vi "仁科参数写入.vi"(11 "簇":T1 {"时间 16"."分钟" format="%.0f分"; "时间 16"."小时" format="%.0f点"; "时间 15"."分钟" format="%.0f分"; "时间 15"."小时" format="%.0f点"; "时间 14"."分钟" format="%.0f分"; "时间 14"."小时" format="%.0f点"; "时间 13"."分钟" format="%.0f分"; "时间 13"."小时" format="%.0f点"; "时间 12"."分钟" format="%.0f分"; "时间 12"."小时" format="%.0f点"; "时间 11"."分钟" format="%.0f分"; "时间 11"."小时" format="%.0f点"; "时间 10"."分钟" format="%.0f分"; "时间 10"."小时" format="%.0f点"; "时间 9"."分钟" format="%.0f分"; "时间 9"."小时" format="%.0f点"; "时间 8"."分钟" format="%.0f分"; "时间 8"."小时" format="%.0f点"; "时间 7"."分钟" format="%.0f分"; "时间 7"."小时" format="%.0f点"; "时间 6"."分钟" format="%.0f分"; "时间 6"."小时" format="%.0f点"; "时间 5"."分钟" format="%.0f分"; "时间 5"."小时" format="%.0f点"; "时间 4"."分钟" format="%.0f分"; "时间 4"."小时" format="%.0f点"; "时间 3"."分钟" format="%.0f分"; "时间 3"."小时" format="%.0f点"; "时间 2"."分钟" format="%.0f分"; "时间 2"."小时" format="%.0f点"; "时间"."分钟" format="%.0f分"; "时间"."小时" format="%.0f点"}) -> (2 "error out":errorcluster)   [LabVIEW 2016, in "环境动力监测库.lvlib" / "空调库.lvlib"]
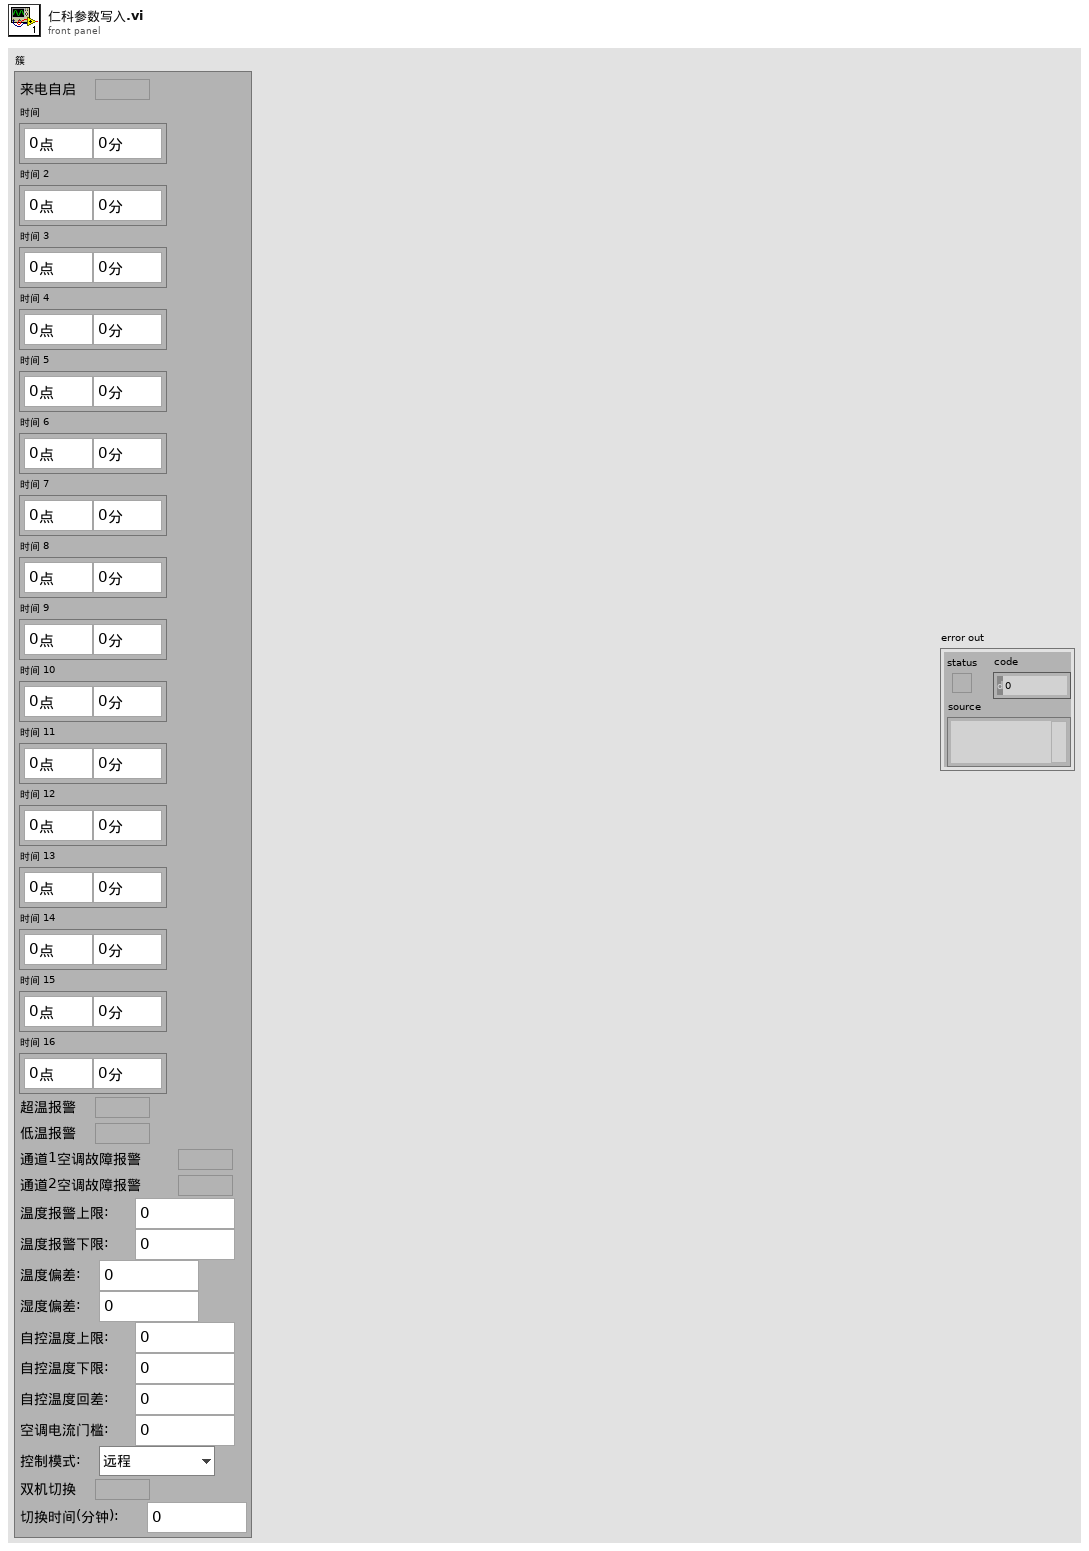
[diagram p1: front panel]
types:
  T1 = cluster{"来电自启":bool, "时间":cluster{"小时":u16, "分钟":u16}, "时间 2":cluster{"小时":u16, "分钟":u16}, "时间 3":cluster{"小时":u16, "分钟":u16}, "时间 4":cluster{"小时":u16, "分钟":u16}, "时间 5":cluster{"小时":u16, "分钟":u16}, "时间 6":cluster{"小时":u16, "分钟":u16}, "时间 7":cluster{"小时":u16, "分钟":u16}, "时间 8":cluster{"小时":u16, "分钟":u16}, "时间 9":cluster{"小时":u16, "分钟":u16}, "时间 10":cluster{"小时":u16, "分钟":u16}, "时间 11":cluster{"小时":u16, "分钟":u16}, "时间 12":cluster{"小时":u16, "分钟":u16}, "时间 13":cluster{"小时":u16, "分钟":u16}, "时间 14":cluster{"小时":u16, "分钟":u16}, "时间 15":cluster{"小时":u16, "分钟":u16}, "时间 16":cluster{"小时":u16, "分钟":u16}, "超温报警":bool, "低温报警":bool, "通道1空调故障报警":bool, "通道2空调故障报警":bool, "温度报警上限:":dbl, "温度报警下限:":dbl, "温度偏差:":dbl, "湿度偏差:":dbl, "自控温度上限:":dbl, "自控温度下限:":dbl, "自控温度回差:":dbl, "空调电流门槛:":dbl, "控制模式:":enum16{"远程", "自动"}, "双机切换":bool, "切换时间(分钟):":dbl}
  T2 = enum16{"open", "read", "write single", "write", "close"}
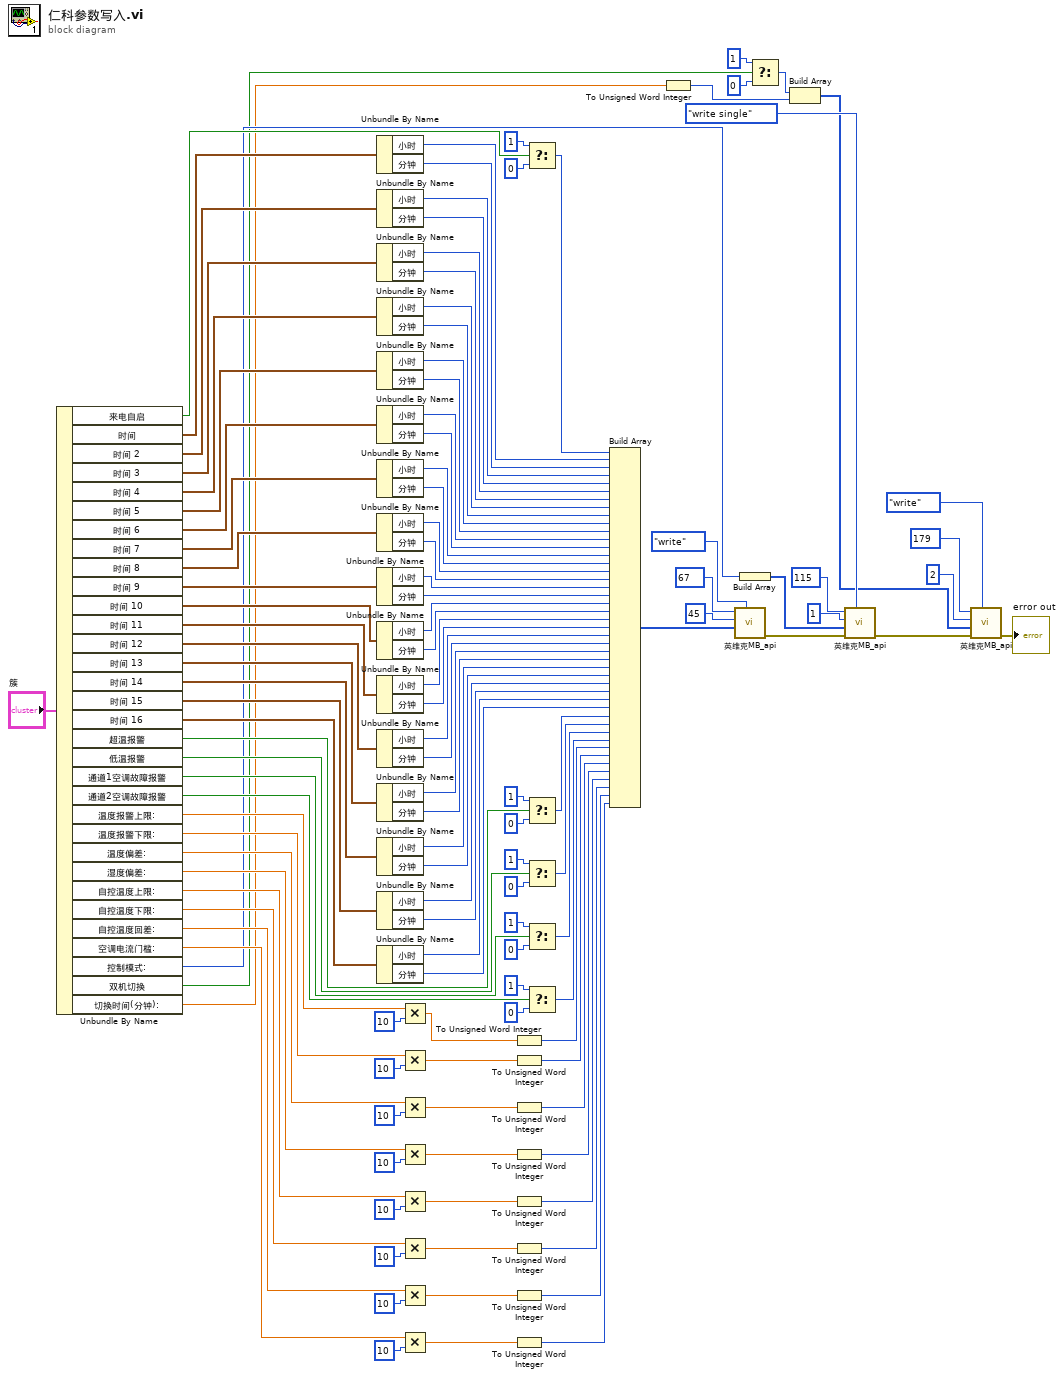
[diagram p0: block diagram]
diagram:
  n1 = Unbundle By Name("簇") -> ("来电自启"=w111:bool, "时间"=w107:cluster{"小时":u16, "分钟":u16}, "时间 2"=w104:cluster{"小时":u16, "分钟":u16}, "时间 3"=w99:cluster{"小时":u16, "分钟":u16}, "时间 4"=w98:cluster{"小时":u16, "分钟":u16}, "时间 5"=w97:cluster{"小时":u16, "分钟":u16}, "时间 6"=w96:cluster{"小时":u16, "分钟":u16}, "时间 7"=w95:cluster{"小时":u16, "分钟":u16}, "时间 8"=w94:cluster{"小时":u16, "分钟":u16}, "时间 9"=w93:cluster{"小时":u16, "分钟":u16}, "时间 10"=w92:cluster{"小时":u16, "分钟":u16}, "时间 11"=w91:cluster{"小时":u16, "分钟":u16}, "时间 12"=w90:cluster{"小时":u16, "分钟":u16}, "时间 13"=w89:cluster{"小时":u16, "分钟":u16}, "时间 14"=w88:cluster{"小时":u16, "分钟":u16}, "时间 15"=w87:cluster{"小时":u16, "分钟":u16}, "时间 16"=w86:cluster{"小时":u16, "分钟":u16}, "超温报警"=w56:bool, "低温报警"=w48:bool, "通道1空调故障报警"=w47:bool, "通道2空调故障报警"=w46:bool, "温度报警上限:"=w40:dbl, "温度报警下限:"=w23:dbl, "温度偏差:"=w22:dbl, "湿度偏差:"=w21:dbl, "自控温度上限:"=w20:dbl, "自控温度下限:"=w19:dbl, "自控温度回差:"=w18:dbl, "空调电流门槛:"=w17:dbl, "控制模式:"=w9:enum16{"远程", "自动"}, "双机切换"=w5:bool, "切换时间(分钟):"=w3:dbl)
  n2 = Unbundle By Name(w107) -> ("小时"=w106:u16, "分钟"=w105:u16)
  n3 = Unbundle By Name(w104) -> ("小时"=w103:u16, "分钟"=w102:u16)
  n4 = Unbundle By Name(w99) -> ("小时"=w85:u16, "分钟"=w84:u16)
  n5 = Unbundle By Name(w98) -> ("小时"=w83:u16, "分钟"=w82:u16)
  n6 = Unbundle By Name(w97) -> ("小时"=w81:u16, "分钟"=w80:u16)
  n7 = Unbundle By Name(w96) -> ("小时"=w79:u16, "分钟"=w78:u16)
  n8 = Unbundle By Name(w95) -> ("小时"=w77:u16, "分钟"=w76:u16)
  n9 = Unbundle By Name(w94) -> ("小时"=w75:u16, "分钟"=w74:u16)
  n10 = Unbundle By Name(w93) -> ("小时"=w73:u16, "分钟"=w72:u16)
  n11 = Unbundle By Name(w92) -> ("小时"=w71:u16, "分钟"=w70:u16)
  n12 = Unbundle By Name(w91) -> ("小时"=w69:u16, "分钟"=w68:u16)
  n13 = Unbundle By Name(w90) -> ("小时"=w67:u16, "分钟"=w66:u16)
  n14 = Unbundle By Name(w89) -> ("小时"=w65:u16, "分钟"=w64:u16)
  n15 = Unbundle By Name(w88) -> ("小时"=w63:u16, "分钟"=w62:u16)
  n16 = Unbundle By Name(w87) -> ("小时"=w61:u16, "分钟"=w60:u16)
  n17 = Unbundle By Name(w86) -> ("小时"=w59:u16, "分钟"=w58:u16)
  n18 = Multiply(x=w40, y=u16 10) -> (x*y=w39:dbl)
  n19 = Multiply(x=w23, y=u16 10) -> (x*y=w37:dbl)
  n20 = Multiply(x=w22, y=u16 10) -> (x*y=w34:dbl)
  n21 = Multiply(x=w21, y=u16 10) -> (x*y=w33:dbl)
  n22 = Multiply(x=w20, y=u16 10) -> (x*y=w25:dbl)
  n23 = Multiply(x=w19, y=u16 10) -> (x*y=w26:dbl)
  n24 = Multiply(x=w18, y=u16 10) -> (x*y=w29:dbl)
  n25 = Multiply(x=w17, y=u16 10) -> (x*y=w30:dbl)
  n26 = To Unsigned Word Integer(number=w39) -> (unsigned 16bit integer=w38:u16)
  n27 = To Unsigned Word Integer(number=w37) -> (unsigned 16bit integer=w16:u16)
  n28 = To Unsigned Word Integer(number=w34) -> (unsigned 16bit integer=w15:u16)
  n29 = To Unsigned Word Integer(number=w33) -> (unsigned 16bit integer=w14:u16)
  n30 = To Unsigned Word Integer(number=w25) -> (unsigned 16bit integer=w13:u16)
  n31 = To Unsigned Word Integer(number=w26) -> (unsigned 16bit integer=w12:u16)
  n32 = To Unsigned Word Integer(number=w29) -> (unsigned 16bit integer=w11:u16)
  n33 = To Unsigned Word Integer(number=w30) -> (unsigned 16bit integer=w10:u16)
  n34 = Select(t=u16 1 ("quantity"), s=w111, f=u16 0 ("quantity")) -> (s? t:f=w108:u16)
  n35 = Select(t=u16 1 ("quantity"), s=w56, f=u16 0 ("quantity")) -> (s? t:f=w45:u16)
  n36 = Select(t=u16 1 ("quantity"), s=w48, f=u16 0 ("quantity")) -> (s? t:f=w44:u16)
  n37 = Select(t=u16 1 ("quantity"), s=w47, f=u16 0 ("quantity")) -> (s? t:f=w43:u16)
  n38 = Select(t=u16 1 ("quantity"), s=w46, f=u16 0 ("quantity")) -> (s? t:f=w42:u16)
  n39 = Build Array(w108, w106, w105, w103, w102, w85, w84, w83, w82, w81, w80, w79, w78, w77, w76, w75, w74, w73, w72, w71, w70, w69, w68, w67, w66, w65, w64, w63, w62, w61, w60, w59, w58, w45, w44, w43, w42, w38, w16, w15, w14, w13, w12, w11, w10) -> (w100:u16[])
  n40 = To Unsigned Word Integer(number=w3) -> (unsigned 16bit integer=w2:u16)
  n41 = call "英维克MB_api.vi"("STEP"=T2."write", "values"=w100, "quantity"=u16 45, "starting address"=u16 67) -> ("error out"=w118:errorcluster)  [unwired: 5 in, 2 out]
  n42 = Build Array(w9) -> (w8:enum16{"远程", "自动"}[])
  n43 = Select(t=u16 1 ("quantity"), s=w5, f=u16 0 ("quantity")) -> (s? t:f=w4:u16)
  n44 = Build Array(w4, w2) -> (w1:u16[])
  n45 = call "英维克MB_api.vi"("STEP"=T2."write single", "Error in"=w118, "values"=w8, "quantity"=u16 1, "starting address"=u16 115) -> ("error out"=w114:errorcluster)  [unwired: 4 in, 2 out]
  n46 = call "英维克MB_api.vi"("STEP"=T2."write", "Error in"=w114, "values"=w1, "quantity"=u16 2, "starting address"=u16 179) -> ("error out"=→"error out":errorcluster)  [unwired: 4 in, 2 out]
